vi "S7Com_REQ(SubVI).vi"(3 "Write Data":T8, 4 "Sequence#":u16, 5 "RW_CMD":T2={"Read Length"=1, "Data Block #"=1, "S7_Add_Area"=132, "Start Address"=0, "S7_Transport_Size"=2, "S7_Function"=4} {"S7_Function" items=["Read"=4, "Write"=5]; "S7_Transport_Size" items=["BIT"=1, "BYTE"=2, "CHAR"=3, "WORD"=4, "INT"=5, "DWORD"=6, "DINT"=7, "REAL"=8]; "S7_Add_Area" items=["P Area"=128, "I Area"=129, "O Area"=130, "M Area"=131, "DB Area"=132, "Counter"=40, "Timer"=41]}) -> (0 "Out Data":T6 format="X%02x", 2 "S7_Transport_Size":T1 items=["BIT"=1, "BYTE"=2, "CHAR"=3, "WORD"=4, "INT"=5, "DWORD"=6, "DINT"=7, "REAL"=8])   [LabVIEW 2019]
doc: "Forms the S7 Protocol Data Request."
uses:
  S7Com_Data_Array.ctl
  S7Com_HexByteArray.ctl
  S7Com_HexByte.ctl
  S7Com_RW_CMD.ctl
  S7Com_Address_Area.ctl
  S7Com_Start_Add.ctl
  S7Com_Transport_Size.ctl
  S7Com_Function.ctl
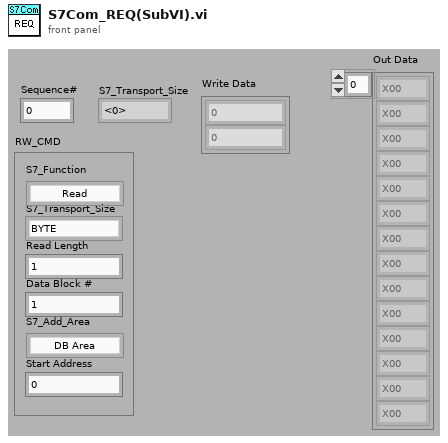
[diagram p1: front panel]
types:
  T1 = typedef "S7Com_Transport_Size.ctl" = u8
  T2 = typedef "S7Com_RW_CMD.ctl" = cluster{"Read Length":u16, "Data Block #":u16, "S7_Add_Area":T3, "Start Address":T4, "S7_Transport_Size":T1, "S7_Function":T5}
  T3 = typedef "S7Com_Address_Area.ctl" = u8
  T4 = typedef "S7Com_Start_Add.ctl" = u16
  T5 = typedef "S7Com_Function.ctl" = u8
  T6 = typedef "S7Com_HexByteArray.ctl" = T7[]
  T7 = typedef "S7Com_HexByte.ctl" = u8
  T8 = typedef "S7Com_Data_Array.ctl" = i32[]
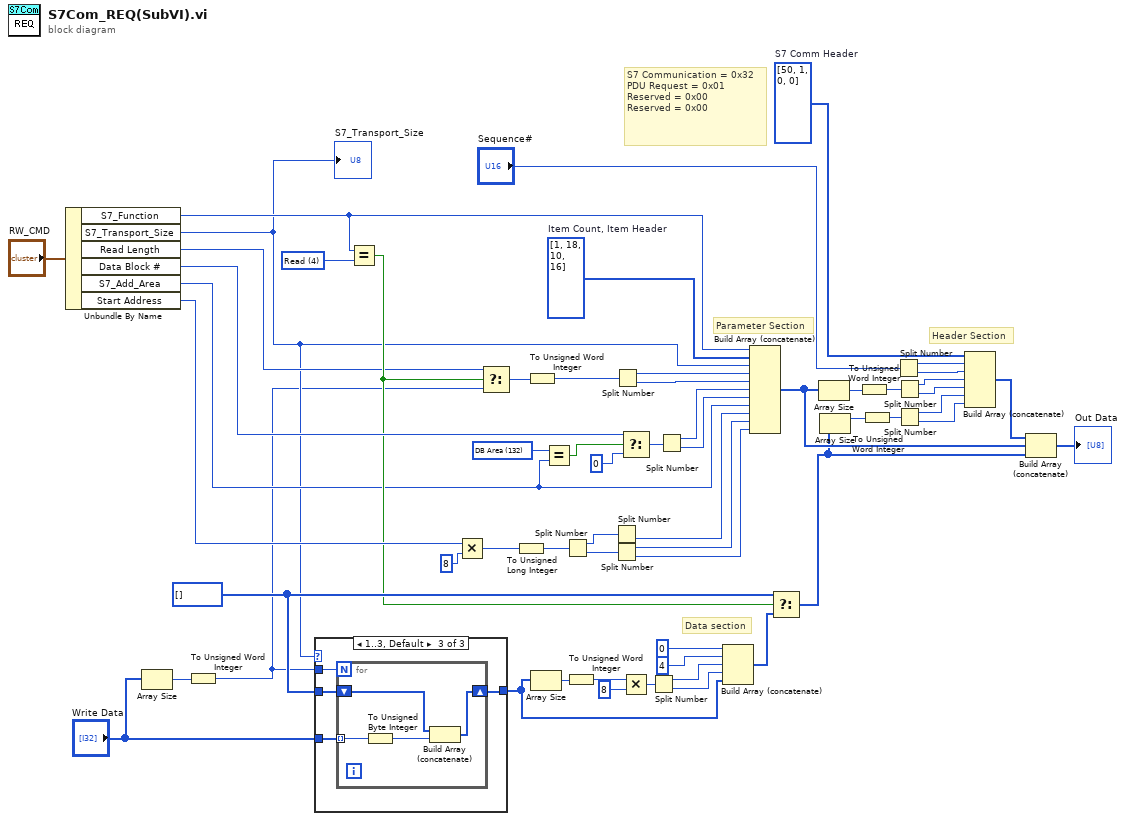
[diagram p0: block diagram]
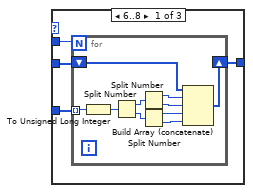
[diagram p2: hidden frame]
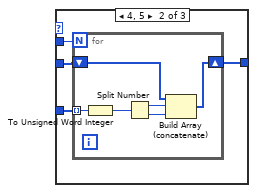
[diagram p3: hidden frame]
diagram:
  w15 = T6 [] ("S7_HexByte_Array")
  w26 = T5 4 items=["Read"=4, "Write"=5] ("S7_Function")
  w51 = T3 132 items=["P Area"=128, "I Area"=129, "O Area"=130, "M Area"=131, "DB Area"=132, "Counter"=40, "Timer"=41] ("S7_Add_Area")
  w33 = u8[] [1, 18, 10, 16]  # Item Count, Item Header
  w57 = u8[] [50, 1, 0, 0]  # S7 Comm Header
  # "Header Section"
  # "Parameter Section"
  # "Data section"
  # "S7 Communication = 0x32\nPDU Request = 0x01\nReserved = 0x00\nReserved = 0x00"
  n1 = Unbundle By Name("RW_CMD") -> ("S7_Function"=w13:T5, "S7_Transport_Size"=w2:T1, "Read Length"=w8:u16, "Data Block #"=w12:u16, "S7_Add_Area"=w7:T3, "Start Address"=w11:T4)
  "S7_Transport_Size" <- w2
  n2 = Array Size(array="Write Data") -> (size(s)=w6:i32)
  n3 = To Unsigned Word Integer(number=w6) -> (unsigned 16bit integer=w1:u16)
  n4 = case shown="1..3, Default" w2 {
    tunnel: [w62 w76 w86] -> w17
    tunnel: "Write Data" -> [w61 w75 w84]
    tunnel: w15 -> [w60 w74 w85]
    tunnel: w1 -> [w59 w73 w83]
    frame 6..8 {
      n5 = for {
        N: w59 -> [_]
        tunnel: w61 -> [w64] mode=indexing
        shift-right: [w72] -> w62
        shift-left: w60 -> [w63]
        n6 = To Unsigned Long Integer(number=w64) -> (unsigned 32bit integer=w65:u32)
        n7 = Split Number(x=w65) -> (hi(x)=w71:u16, lo(x)=w70:u16)
        n8 = Split Number(x=w71) -> (hi(x)=w69:u8, lo(x)=w68:u8)
        n9 = Split Number(x=w70) -> (hi(x)=w66:u8, lo(x)=w67:u8)
        n10 = Build Array (concatenate)(w63, w69, w68, w66, w67) -> (w72:T6)
      }
    }
    frame 4, 5 {
      n11 = for {
        N: w73 -> [_]
        tunnel: w75 -> [w78] mode=indexing
        shift-right: [w82] -> w76
        shift-left: w74 -> [w77]
        n12 = To Unsigned Word Integer(number=w78) -> (unsigned 16bit integer=w79:u16)
        n13 = Split Number(x=w79) -> (hi(x)=w81:u8, lo(x)=w80:u8)
        n14 = Build Array (concatenate)(w77, w81, w80) -> (w82:T6)
      }
    }
    frame 1..3, Default {
      n15 = for {
        N: w83 -> [_]
        shift-right: [w90] -> w86
        shift-left: w85 -> [w89]
        tunnel: w84 -> [w88] mode=indexing
        n16 = To Unsigned Byte Integer(number=w88) -> (unsigned 8bit integer=w87:u8)
        n17 = Build Array (concatenate)(w89, w87) -> (w90:T6)
      }
    }
  }
  n18 = Equal?(x=w13, y=w26) -> (x = y?=w10:bool)
  n19 = Multiply(x=w11, y=T4 8) -> (x*y=w5:T4)
  n20 = Select(t=w8, s=w10, f=w1) -> (s? t:f=w9:u16)
  n21 = To Unsigned Long Integer(number=w5) -> (unsigned 32bit integer=w4:u32)
  n22 = To Unsigned Word Integer(number=w9) -> (unsigned 16bit integer=w3:u16)
  n23 = Array Size(array=w17) -> (size(s)=w48:i32)
  n24 = Equal?(x=w51, y=w7) -> (x = y?=w52:bool)
  n25 = Split Number(x=w4) -> (hi(x)=w35:u16, lo(x)=w34:u16)
  n26 = To Unsigned Word Integer(number=w48) -> (unsigned 16bit integer=w18:u16)
  n27 = Split Number(x=w35) -> (lo(x)=w21:u8)  [unwired: 1 out]
  n28 = Split Number(x=w34) -> (hi(x)=w22:u8, lo(x)=w23:u8)
  n29 = Split Number(x=w3) -> (hi(x)=w30:u8, lo(x)=w31:u8)
  n30 = Select(t=w12, s=w52, f=u16 0) -> (s? t:f=w55:u16)
  n31 = Multiply(x=w18, y=u16 8) -> (x*y=w19:u16)
  n32 = Split Number(x=w19) -> (hi(x)=w45:u8, lo(x)=w44:u8)
  n33 = Split Number(x=w55) -> (hi(x)=w54:u8, lo(x)=w53:u8)
  n34 = Build Array (concatenate)(u8 0, u8 4, w45, w44, w17) -> (w24:T6)
  n35 = Build Array (concatenate)(w13, w33, w2, w30, w31, w54, w53, w7, w21, w22, w23) -> (w28:T3[])
  n36 = Select(t=w15, s=w10, f=w24) -> (s? t:f=w25:T6)
  n37 = Array Size(array=w28) -> (size(s)=w32:i32)
  n38 = Array Size(array=w25) -> (size(s)=w43:i32)
  n39 = To Unsigned Word Integer(number=w32) -> (unsigned 16bit integer=w40:u16)
  n40 = To Unsigned Word Integer(number=w43) -> (unsigned 16bit integer=w37:u16)
  n41 = Split Number(x="Sequence#") -> (hi(x)=w50:u8, lo(x)=w49:u8)
  n42 = Split Number(x=w40) -> (hi(x)=w42:u8, lo(x)=w41:u8)
  n43 = Split Number(x=w37) -> (hi(x)=w39:u8, lo(x)=w38:u8)
  n44 = Build Array (concatenate)(w57, w50, w49, w42, w41, w39, w38) -> (w29:u8[])
  n45 = Build Array (concatenate)(w29, w28, w25) -> (→"Out Data":T6)
